vi "FRCts20_Backend_Stats_Reform_RequestsPerHour.vi"(8 "error in (no error)":errorcluster, 11 "Array":T1(array[cluster])) -> (0 "Error Out":errorcluster, 3 "RequestsPerHour":T2)   [LabVIEW 2014, in "FRCts20_Backend_Engine.lvlib"]
uses:
  FRCts20_Backend_Engine.lvlib
  ESP Engine/source/VI Source/TypeDefs/FRCts20_EspEngine_RequestPerHour_Line.ctl
  FRCts20_Backend_API/FRCts20_Backend_API_Stats.ctl
  ESP Engine/source/VI Source/TypeDefs/FRCts20_EspEngine_SwUsage_Pie.ctl
  ESP Engine/source/VI Source/TypeDefs/FRCts20_EspEngine_AdvancedComponents_Bar.ctl
  ESP Engine/source/VI Source/FRCts20_EspEngine.lvlib
  FRCts20_Backend_API/FRCts20_Backend_API.lvlib
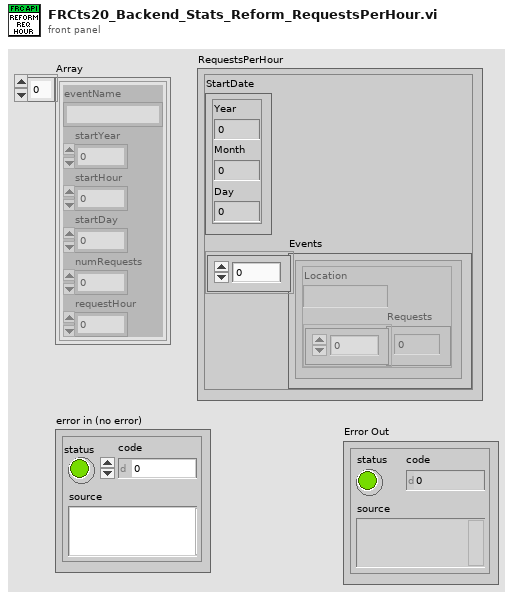
[diagram p1: front panel]
types:
  T1 = cluster{"eventName":string, "startYear":i32, "startHour":i32, "startDay":i32, "numRequests":i32, "requestHour":i32}[]
  T2 = typedef "FRCts20_EspEngine.lvlib/FRCts20_EspEngine_RequestPerHour_Line.ctl" = cluster{"StartDate":cluster{"Year":i32, "Month":i32, "Day":i32}, "Events":cluster{"Location":string, "Requests":i32[]}[]}
  T3 = typedef "FRCts20_Backend_Engine.lvlib/FRCts20_Backend_API.lvlib/FRCts20_Backend_API_Stats.ctl" = cluster{"RequestsPerHour":T2, "SW Usage Pies":T4, "Advanced Components":T5, "APIReturn":string}
  T4 = typedef "FRCts20_EspEngine.lvlib/FRCts20_EspEngine_SwUsage_Pie.ctl" = cluster{"Live Event Location":string, "LabVIEW":dbl, "C++":dbl, "Java":dbl, "Other":dbl, "TotalTeams":i32, "TeamsReporting":i32}[]
  T5 = typedef "FRCts20_EspEngine.lvlib/FRCts20_EspEngine_AdvancedComponents_Bar.ctl" = cluster{"CAN":i32, "Vision":i32, "Kinect":i32}
  T6 = cluster{"eventName":string, "startYear":i32, "startHour":i32, "startDay":i32, "numRequests":i32, "requestHour":i32}
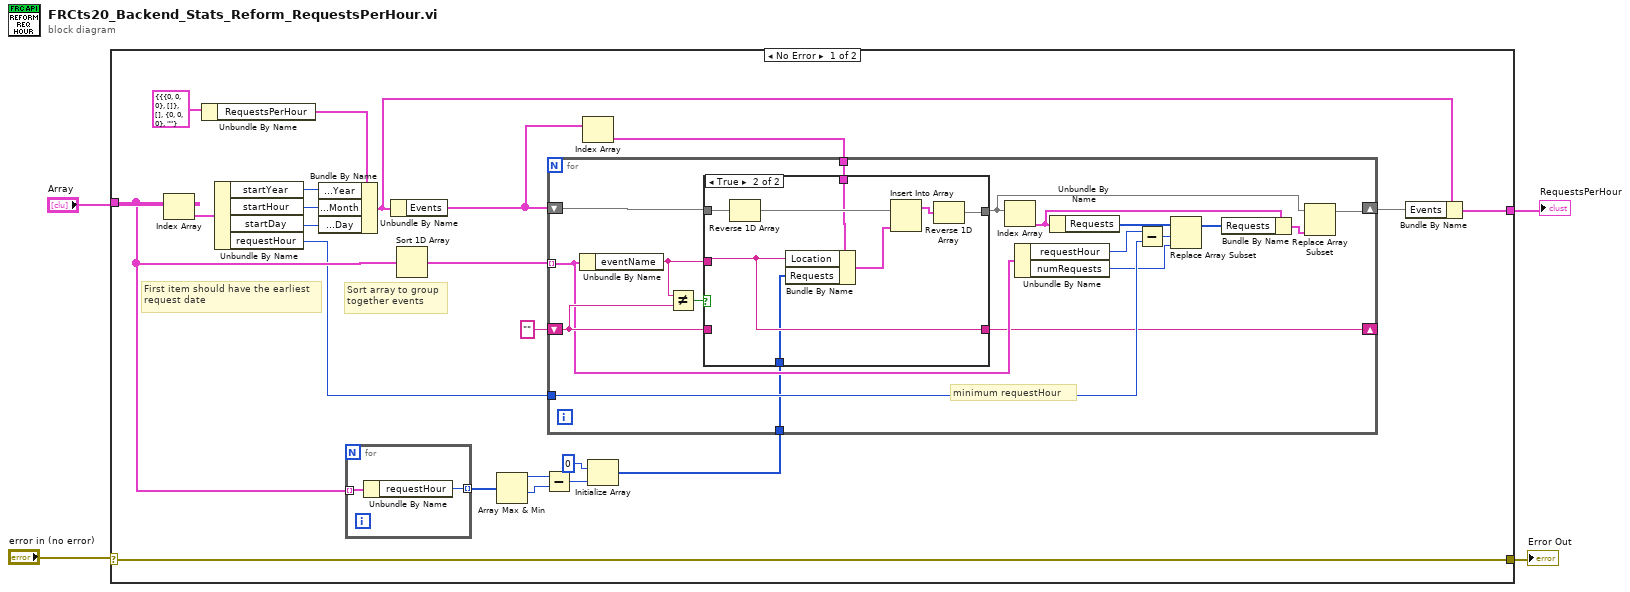
[diagram p0: block diagram]
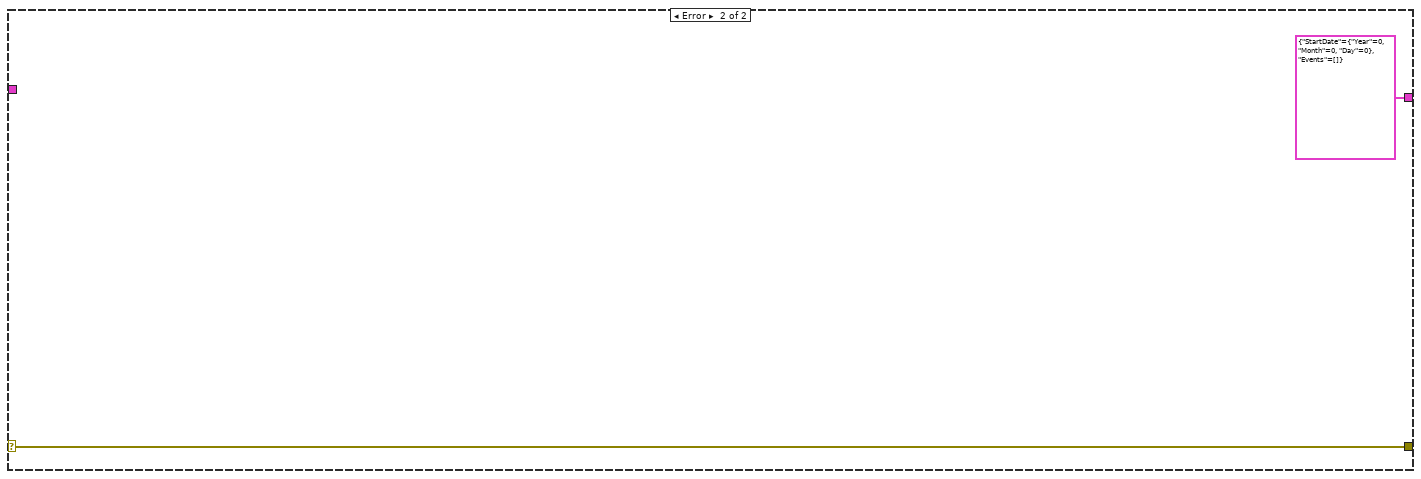
[diagram p3: hidden frame]
diagram:
  n1 = case shown="No Error" "error in (no error)" {
    selector: "error in (no error)" -> [w26 w57]
    tunnel: "Array" -> [w16 _]
    tunnel: [w26 w57] -> w3
    tunnel: [w5 T2 {"StartDate"={"Year"=0, "Month"=0, "Day"=0}, "Events"=[]} ("RequestsPerHour")] -> w1
    frame No Error {
      # "Sort array to group\ntogether events"
      # "First item should have the earliest\nrequest date"
      n2 = Index Array(array=w16) -> (element=w25:T6)  [unwired: 1 in]
      n3 = Unbundle By Name(T3 {"RequestsPerHour"={"StartDate"={"Year"=0, "Month"=0, "Day"=0}, "Events"=[]}, "SW Usage Pies"=[], "Advanced Components"={"CAN"=0, "Vision"=0, "Kinect"=0}, "APIReturn"=""} ("Statistics")) -> ("RequestsPerHour"=w20:T2)
      n4 = Unbundle By Name(w25) -> ("startYear"=w23:i32, "startHour"=w22:i32, "startDay"=w21:i32, "requestHour"=w14:i32)
      n5 = Bundle By Name(cluster=w20, "StartDate.Year"=w23, "StartDate.Month"=w22, "StartDate.Day"=w21) -> (w7:T2)
      n6 = for {
        tunnel: w16 -> [w28] mode=indexing
        tunnel: [w27] -> w15 mode=indexing
        n7 = Unbundle By Name(w28) -> ("requestHour"=w27:i32)
      }
      n8 = Unbundle By Name(w7) -> ("Events"=w11:cluster{"Location":string, "Requests":i32[]}[])
      n9 = Sort 1D Array(array=w16) -> (sorted array=w17:T1)
      n10 = Array Max & Min(array=w15) -> (max value=w13:i32, min value=w12:i32)  [unwired: 2 out]
      n11 = Subtract(x=w13, y=w12) -> (x-y=w10:i32)
      n12 = Index Array(array=w11) -> (element=w18:cluster{"Location":string, "Requests":i32[]})  [unwired: 1 in]
      n13 = Initialize Array(0 ("element"), w10) -> (w8:i32[])
      n14 = for {
        shift-right: [w41] -> w6
        shift-left: w11 -> [w43]
        shift-right: [w30] -> _
        shift-left: "" -> [w45]
        tunnel: w17 -> [w42] mode=indexing
        tunnel: w18 -> [w44]
        tunnel: w14 -> [w38]
        tunnel: w8 -> [w37]
        # "minimum requestHour"
        n15 = Unbundle By Name(w42) -> ("eventName"=w29:string)
        n16 = Not Equal?(x=w29, y=w45) -> (x != y?=w46:bool)
        n17 = case shown="True" w46 {
          tunnel: [w47 w54] -> w40
          tunnel: w45 -> [w48 _]
          tunnel: [w48 w50] -> w30
          tunnel: w29 -> [_ w50]
          tunnel: w44 -> [_ w53]
          tunnel: w43 -> [w47 w52]
          tunnel: w37 -> [_ w49]
          frame False {
          }
          frame True {
            n18 = Reverse 1D Array(array=w52) -> (reversed array=w56:cluster{"Location":string, "Requests":i32[]}[])
            n19 = Bundle By Name(cluster=w53, "Location"=w50, "Requests"=w49) -> (w51:cluster{"Location":string, "Requests":i32[]})
            n20 = Insert Into Array(array=w56, new element=w51) -> (w55:cluster{"Location":string, "Requests":i32[]}[])  [unwired: 1 in]
            n21 = Reverse 1D Array(array=w55) -> (reversed array=w54:cluster{"Location":string, "Requests":i32[]}[])
          }
        }
        n22 = Index Array(array=w40) -> (element=w35:cluster{"Location":string, "Requests":i32[]})  [unwired: 1 in]
        n23 = Unbundle By Name(w42) -> ("requestHour"=w39:i32, "numRequests"=w31:i32)
        n24 = Unbundle By Name(w35) -> ("Requests"=w36:i32[])
        n25 = Subtract(x=w39, y=w38) -> (x-y=w32:i32)
        n26 = Replace Array Subset(array=w36, new element=w31, index=w32) -> (w34:i32[])
        n27 = Bundle By Name(cluster=w35, "Requests"=w34) -> (w33:cluster{"Location":string, "Requests":i32[]})
        n28 = Replace Array Subset(array=w40, new element=w33) -> (w41:cluster{"Location":string, "Requests":i32[]}[])  [unwired: 1 in]
      }
      n29 = Bundle By Name(cluster=w7, "Events"=w6) -> (w5:T2)
    }
    frame Error {
    }
  }
  "RequestsPerHour" <- w1
  "Error Out" <- w3
